vi "struct_abs_act_x_pTv1v2.vi"(0 "Reference working pair (Input)":i64, 1 "Molar volume of second component in m3/mol (Input)":dbl, 5 "Pressure p_Pa in Pa (Input)":dbl, 7 "Temperature in K (Input)":dbl, 9 "Molar volume of first component in m3/mol (Input)":dbl, 11 "Error (Input)":errorcluster) -> (4 "Mole fraction in liquid phase in mol/mol (Output)":dbl, 15 "Error (Output)":errorcluster)   [LabVIEW 2017]
doc: "abs_act_x_pTv1v2:\n * -----------------\n *\n * Calculates mole fraction of first component in liquid phase x_molmol in\n * mol/mol depending on equilibrium pressure p_Pa in Pa of first component,\n * temperature T_K in K, molar volume of first component in m³/mol, and molar\n * volume of second component in m³/mol.\n *\n * Parameters:\n * -----------\n * double p_Pa:\n * Equilibrium pressure p_Pa in Pa.\n * double T_K:\n * Equilibrium temperature in K.\n * double v1_m3mol:\n * Equilibrium molar volume of first component in m³/mol.\n * double v2_m3mol:\n * Equilibrium molar volume of second component in m³/mol.\n * struct *WorkingPair:\n * Pointer of WorkingPair-struct.\n *\n * Returns:\n * --------\n * double:\n * Equilibrium mole fraction in liquid phase in mol/mol.\n *\n * Remarks:\n * --------\n * This function is only valid for isotherm models based on activity\n * coefficients.\n * Molar volumes may are not required and ignored. When molar volumes are\n * required, function uses molar volumes stored in JSON file when input\n * v1_m3mol or v2_m3mol is -1. Otherwise, function uses molar volumes given by\n * inputs.\n * This function uses internal model for vapor pressure of refrigerant.\n *\n * History:\n * --------\n * 07/14/2021, by Jannik Driesel (supervised by Mirko Engelpracht):\n * First implementation."
uses:
  data/win32bit/libsorpPropLib.dll
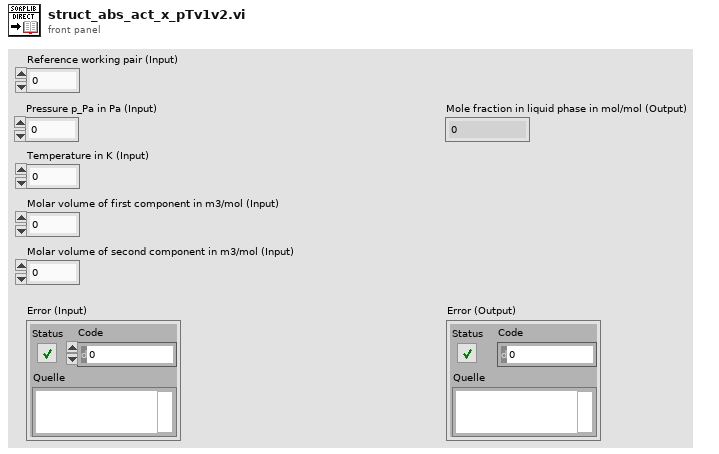
[diagram p1: front panel]
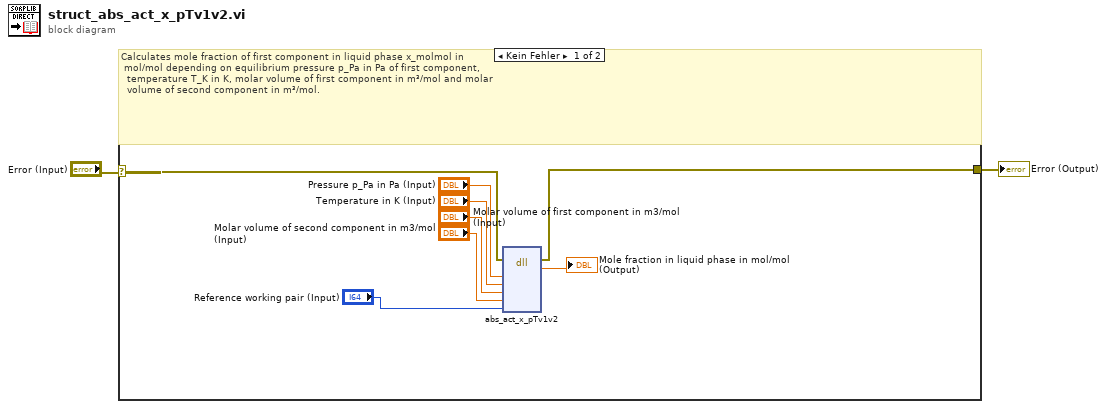
[diagram p0: block diagram]
diagram:
  n1 = case shown="Kein Fehler" "Error (Input)" {
    selector: "Error (Input)" -> [w10 w11]
    tunnel: [w9 w11] -> w2
    frame No Error {
      # "Calculates mole fraction of first component in liquid phase x_molmol in\n mol/mol depending on equilibrium pressure p_Pa in Pa of first component,\n  temperature T_K in K, molar volume of first component in m³/mol and molar\n  volume of second component in m³/mol."
      n2 = dll-call lib="D:/Driesel/SorpLibLocal/LabVIEW_wrapper/data/win32bit/libsorpPropLib.dll" fn="abs_act_x_pTv1v2"(error in=w10, "p_Pa"="Pressure p_Pa in Pa (Input)", "T_K"="Temperature in K (Input)", "v1_m3mol"="Molar volume of first component in m3/mol (Input)", "v2_m3mol"="Molar volume of second component in m3/mol (Input)", "workingPair"="Reference working pair (Input)") -> (error out=w9:errorcluster, "x_molmol"=→"Mole fraction in liquid phase in mol/mol (Output)":dbl)  [unwired: 7 in, 1 out]
    }
    frame Error {
      # "Error - No calculations"
    }
  }
  "Error (Output)" <- w2
